vi "Run.vi"(11 "SettingsFile in":refnum<class "SettingsFile.lvclass">) -> (3 "SettingsFile out":refnum<class "SettingsFile.lvclass">)   [LabVIEW 2018, in "SettingsFile.lvclass"]
uses:
  SettingsFile.lvclass
  SettingsFile.lvclass/SettingsFile.ctl
  Communication/global_stop.vi
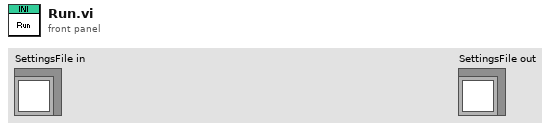
[diagram p1: front panel]
types:
  T1 = typedef "INI Save Event.ctl" = refnum<user-event>
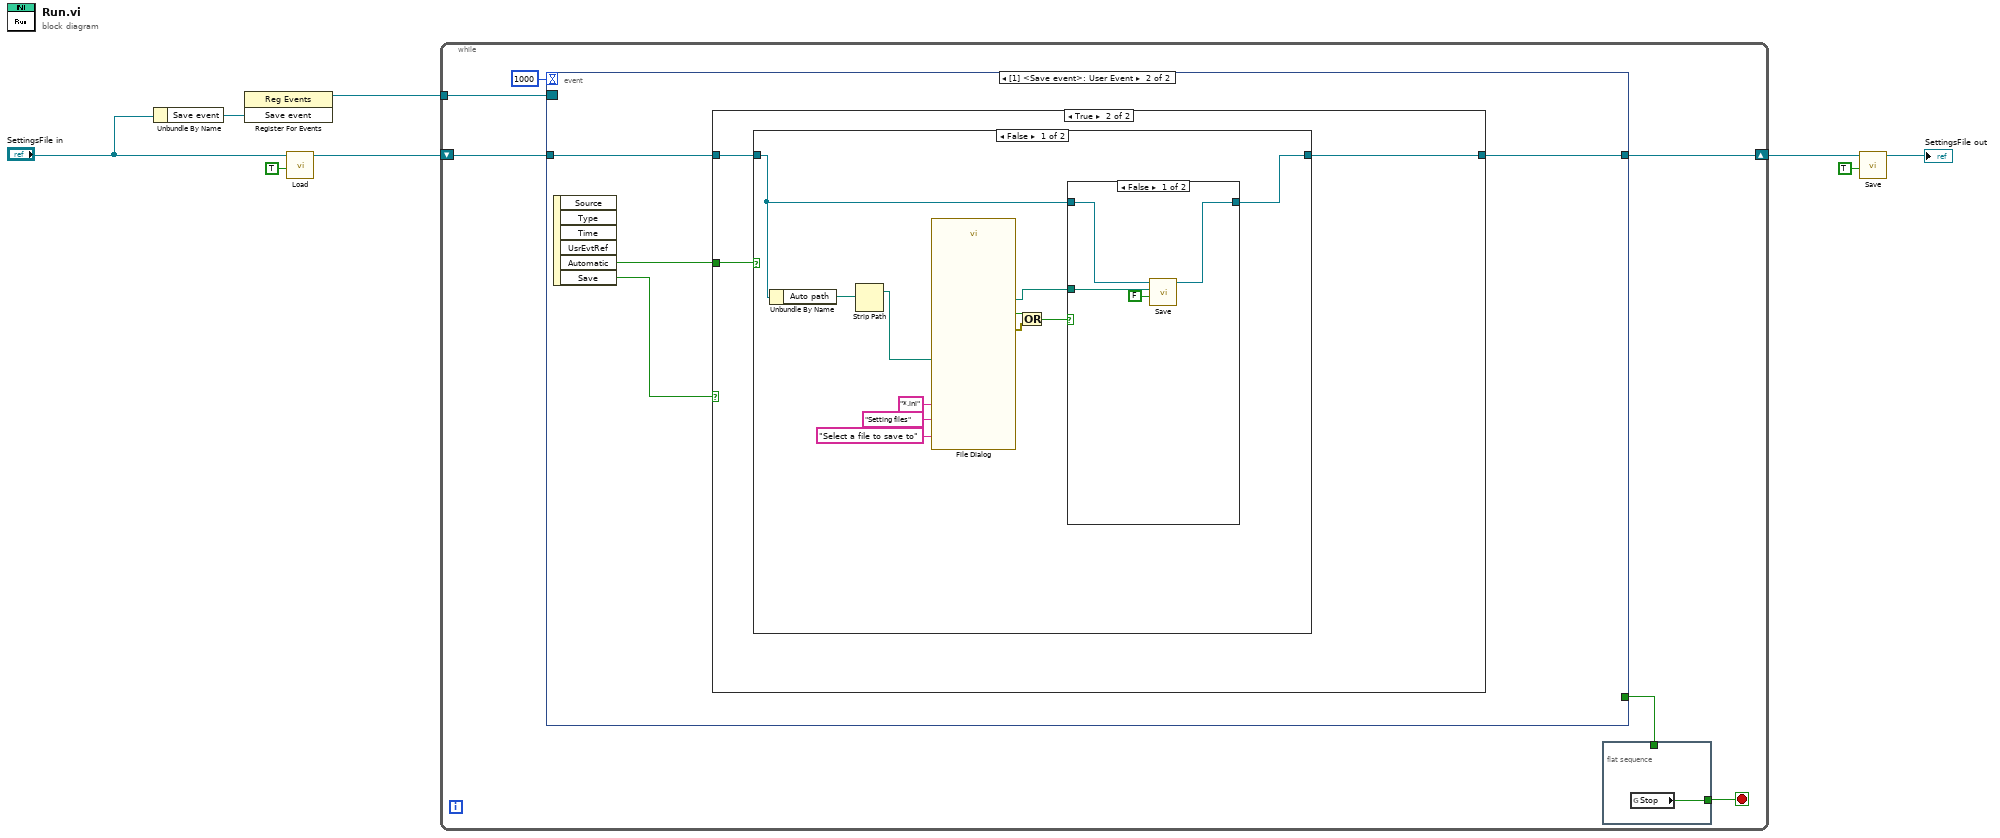
[diagram p0: block diagram]
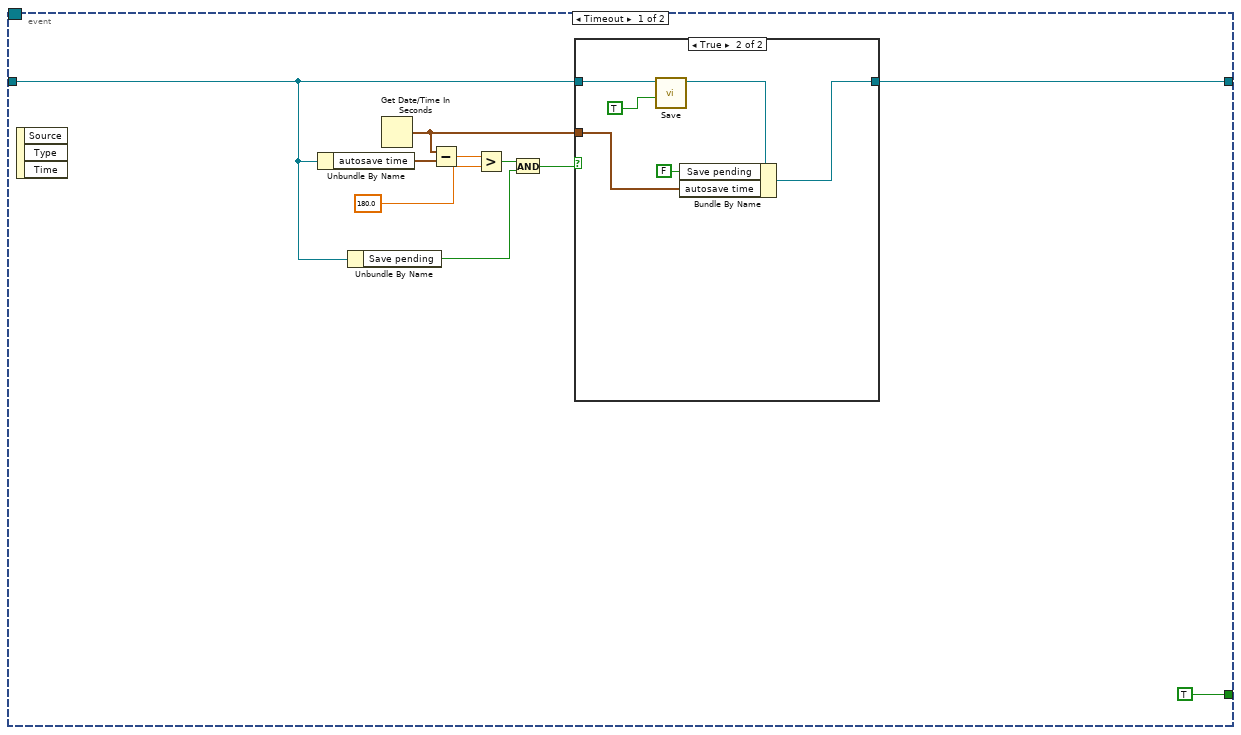
[diagram p2: hidden frame]
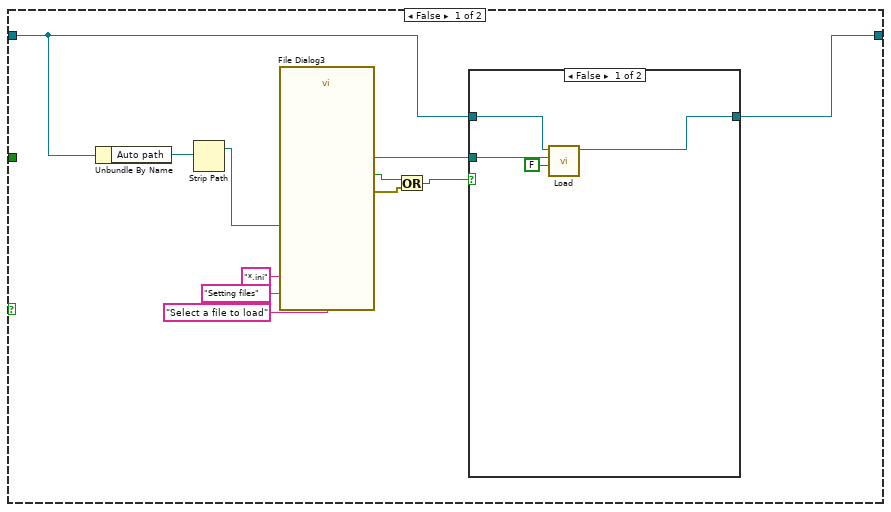
[diagram p4: hidden frame]
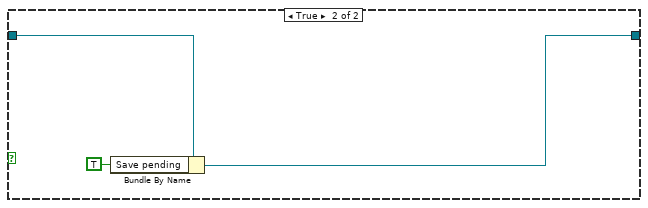
[diagram p7: hidden frame]
diagram:
  n1 = Unbundle By Name("SettingsFile in") -> ("Save event"=w7:T1)
  n2 = register-events(w7) -> (reference out=w8:refnum<event-registration>)  [unwired: 2 in, 1 out]
  n3 = call "Load.vi"("Automatic?"=TRUE, "SettingsFile in"="SettingsFile in") -> ("SettingsFile out"=w5:refnum<class "SettingsFile.lvclass">)  [unwired: 8 in, 1 out]
  n4 = while {
    shift-right: [w13] -> w3
    shift-left: w5 -> [w14]
    tunnel: w8 -> [w12]
    stop <- w10 stop-if-true
    n5 = event shown="[1] <Save event>: User Event" {
      selector: w12 -> [_ _]
      dyn-events: _ -> [_ _]
      timeout: 1000 -> [_ _]
      tunnel: w14 -> [w21 w36]
      tunnel: [w16 w35] -> w13
      tunnel: [TRUE _] -> w9
      event Timeout {
        n6 = event-data() -> ()  [unwired: 1 in, 3 out]
        n7 = Unbundle By Name(w21) -> ("autosave time"=w24:timestamp)
        n8 = Unbundle By Name(w21) -> ("Save pending"=w19:bool)
        n9 = Get Date/Time In Seconds() -> (seconds since 1Jan1904=w17:timestamp)
        n10 = Subtract(x=w17, y=w24) -> (x-y=w23:dbl)
        n11 = Greater?(x=w23, y=180.0) -> (0:w20:bool)
        n12 = And(x=w20, y=w19) -> (x .and. y?=w18:bool)
        n13 = case shown="True" w18 {
          tunnel: w21 -> [w26 w31]
          tunnel: w17 -> [_ w28]
          tunnel: [w26 w27] -> w16
          frame False {
          }
          frame True {
            n14 = call "Save.vi"("Automatic?"=TRUE, "SettingsFile in"=w31) -> ("SettingsFile out"=w30:refnum<class "SettingsFile.lvclass">)  [unwired: 8 in, 1 out]
            n15 = Bundle By Name(cluster=w30, "Save pending"=FALSE, "autosave time"=w28) -> (w27:refnum<class "SettingsFile.lvclass">)
          }
        }
      }
      event User Event {
        n16 = event-data() -> ("Automatic"=w33:bool, "Save"=w34:bool)  [unwired: 1 in, 4 out]
        n17 = case shown="True" w34 {
          tunnel: w36 -> [w38 w55]
          tunnel: [w37 w53] -> w35
          tunnel: w33 -> [_ w54]
          frame False {
            n18 = Unbundle By Name(w38) -> ("Auto path"=w47:path)
            n19 = Strip Path(path=w47) -> (stripped path=w46:path)  [unwired: 1 out]
            n20 = call "File Dialog3"("start path"=w46, "prompt"="Select a file to load", "pattern (all files)"="*.ini", "pattern label"="Setting files") -> ("selected path"=w40:path, "cancelled"=w42:bool, "error out"=w41:errorcluster)  [unwired: 8 in, 1 out]
            n21 = Or(x=w42, y=w41) -> (x .or. y?=w39:bool)
            n22 = case shown="False" w39 {
              tunnel: w40 -> [w51 _]
              tunnel: w38 -> [w49 w52]
              tunnel: [w48 w52] -> w37
              frame False {
                n23 = call "Load.vi"("Automatic?"=FALSE, "configuration file path"=w51, "SettingsFile in"=w49) -> ("SettingsFile out"=w48:refnum<class "SettingsFile.lvclass">)  [unwired: 7 in, 1 out]
              }
              frame True {
              }
            }
          }
          frame True {
            n24 = case shown="False" w54 {
              tunnel: w55 -> [w58 w74]
              tunnel: [w56 w72] -> w53
              frame False {
                n25 = Unbundle By Name(w58) -> ("Auto path"=w63:path)
                n26 = Strip Path(path=w63) -> (stripped path=w62:path)  [unwired: 1 out]
                n27 = call "File Dialog"("start path"=w62, "prompt"="Select a file to save to", "pattern (all files)"="*.ini", "pattern label"="Setting files") -> ("selected path"=w57:path, "cancelled"=w61:bool, "error out"=w60:errorcluster)  [unwired: 8 in, 1 out]
                n28 = Or(x=w61, y=w60) -> (x .or. y?=w59:bool)
                n29 = case shown="False" w59 {
                  tunnel: w58 -> [w70 w71]
                  tunnel: w57 -> [w69 _]
                  tunnel: [w67 w71] -> w56
                  frame False {
                    n30 = call "Save.vi"("Automatic?"=FALSE, "configuration file path"=w69, "SettingsFile in"=w70) -> ("SettingsFile out"=w67:refnum<class "SettingsFile.lvclass">)  [unwired: 7 in, 1 out]
                  }
                  frame True {
                  }
                }
              }
              frame True {
                n31 = Bundle By Name(cluster=w74, "Save pending"=TRUE) -> (w72:refnum<class "SettingsFile.lvclass">)
              }
            }
          }
        }
      }
    }
    n32 = flat-sequence {
      tunnel: [w15] -> w10
      tunnel: w9 -> [_]
      frame #0 {
        n33 = global read "global_stop.vi" "Stop"() -> (w15:bool)
      }
    }
  }
  n34 = call "Save.vi"("Automatic?"=TRUE, "SettingsFile in"=w3) -> ("SettingsFile out"=→"SettingsFile out":refnum<class "SettingsFile.lvclass">)  [unwired: 8 in, 1 out]
